vi "Test Verify Valid Account.vi"(8 "error in (no error)":errorcluster, 11 "Test Case In":refnum<class "Account Database Test.lvclass">) -> (0 "error out":errorcluster, 3 "Test Case Out":refnum<class "Account Database Test.lvclass">)   [LabVIEW 2020, in "Account Database Test.lvclass"]
uses:
  Account Database Test.lvclass
  C:/Program Files (x86)/National Instruments/LabVIEW 2020/vi.lib/Astemes/LUnit/Test Case.lvclass
  <vilib>/Astemes/LUnit/Test Case.lvclass/Test Case.ctl
  <vilib>/Astemes/LUnit/Palette/Fail.vi
  <vilib>/Astemes/LUnit/Palette/Pass.vi
  <vilib>/Astemes/LUnit/Set Assertion Type.vi
  <vilib>/Astemes/LUnit/Add test result.vi
  <vilib>/Astemes/LUnit/LUnit Record Assertion Result.vi
  <vilib>/Astemes/LUnit/LUnit Aggregate Assertion Results.vi
  <vilib>/Astemes/LUnit/Method Result/LUnit Merge Status.vi
  <vilib>/Astemes/LUnit/LUnit Concatenate result strings.vi
  Account Database Test.lvclass/Account Database Test.ctl
  Account Database/Account Database.lvclass
  <vilib>/Astemes/LUnit/Test Case.lvclass
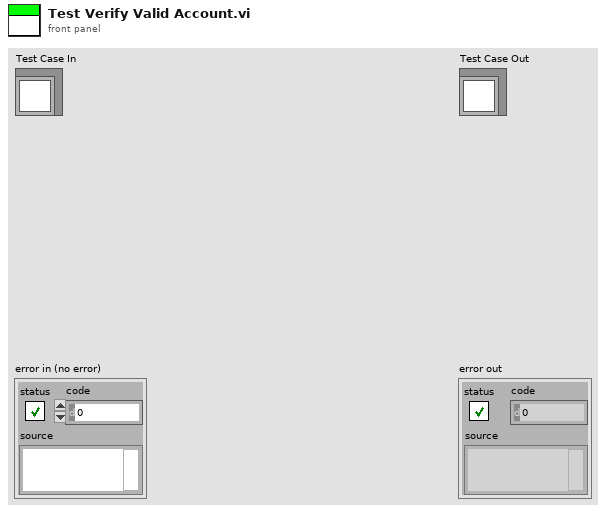
[diagram p1: front panel]
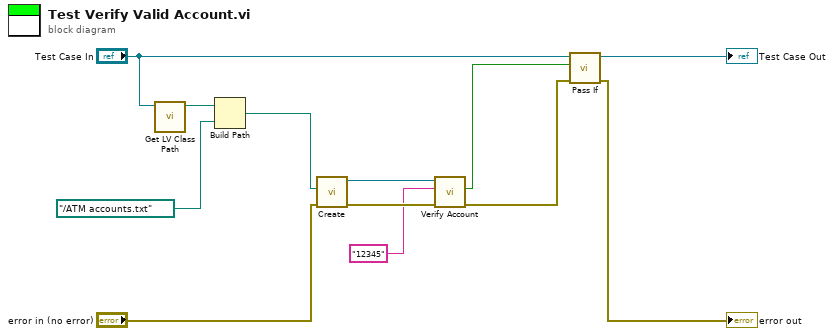
[diagram p0: block diagram]
diagram:
  n1 = call <vilib>:"Get LV Class Path.vi"("object"="Test Case In") -> ("class path"=w9:path)  [unwired: 9 in, 1 out]
  n2 = Build Path(base path=w9, name or relative path=path "../ATM accounts.txt") -> (appended path=w7:path)
  n3 = call "Create.vi"("error in (no error)"="error in (no error)", "Data File"=w7) -> ("error out"=w5:errorcluster, "Account Database out"=w3:refnum<class "Account Database.lvclass">)  [unwired: 8 in]
  n4 = call "Verify Account.vi"("error in (no error)"=w5, "Account Number"="12345", "Account Database in"=w3) -> ("error out"=w4:errorcluster, "Valid Account Number?"=w1:bool)  [unwired: 6 in, 1 out]
  n5 = call <vilib>:"Pass If.vi"("error in (no error)"=w4, "Pass?"=w1, "LUnit Test Case In"="Test Case In") -> ("error out"=→"error out":errorcluster, "LUnit Test Case Out"=→"Test Case Out":refnum<class "Account Database Test.lvclass">)  [unwired: 7 in]
